vi "Destroy.vi"(0 "reference in":refnum<class "GUI Controller.lvclass">, 5 "error in (no error)":errorcluster) -> (14 "reference out":refnum<class "GUI Controller.lvclass">, 19 "error out":errorcluster)   [LabVIEW 2015, in "GUI Controller.lvclass"]
doc: "Destructor."
uses:
  GUI Controller.lvclass
  <vilib>/addons/_AddQ/G#Object/G#Object.lvclass
  Project Panels_class/Project Panels.lvclass
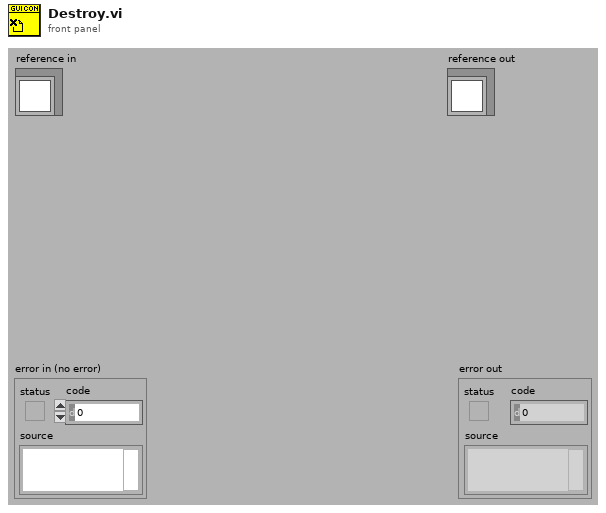
[diagram p1: front panel]
types:
  T1 = typedef "GUI Controller.lvclass/ObjectAttributes.ctl" = cluster{"MyAttribute":dbl, "state":T2, "project_panels_ref":refnum<class "Project Panels.lvclass">, "file_controller_ref":refnum<class "File Controller.lvclass">, "subject_controller_ref":refnum<class "Subject Controller.lvclass">}
  T2 = typedef "GUI Controller.lvclass/state.ctl" = enum16{"initiate", "AddNewFile", "ElaborateData", "CheckData", "waitEvent", "checkSubject", "ChangeSubject", "stop"}
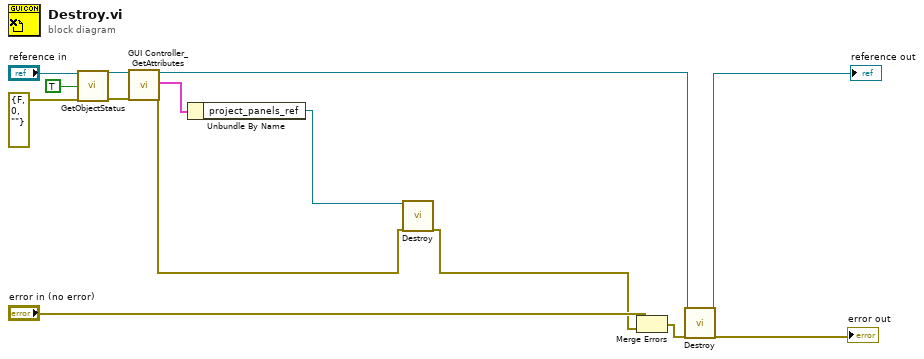
[diagram p0: block diagram]
diagram:
  n1 = call-dynamic "GetObjectStatus.vi"("reference in"="reference in", "simple info (F)"=TRUE ("simple info"), "error in (no error)"=errorcluster {"status"=FALSE, "code"=0, "source"=""}) -> ("reference out"=w8:refnum<class "GUI Controller.lvclass">, "error out"=w9:errorcluster)  [unwired: 5 in, 10 out]
  n2 = call "GUI Controller_GetAttributes.vi"("reference in"=w8, "error in (no error)"=w9) -> ("reference out"=w7:refnum<class "GUI Controller.lvclass">, "attributes"=w6:T1, "error out"=w2:errorcluster)  [unwired: 14 in, 1 out]
  n3 = Unbundle By Name(w6) -> ("project_panels_ref"=w3:refnum<class "Project Panels.lvclass">)
  n4 = call-dynamic "Destroy.vi"("reference in"=w3, "error in (no error)"=w2) -> ("error out"=w1:errorcluster)  [unwired: 16 in, 1 out]
  n5 = Merge Errors("error in (no error)", w1) -> (w13:errorcluster)
  n6 = call-parent "Destroy.vi"("reference in"=w7, "error in (no error)"=w13) -> ("reference out"=→"reference out":refnum<class "GUI Controller.lvclass">, "error out"=→"error out":errorcluster)  [unwired: 16 in]
